vi "MNIST_WB big pattern_LCD_sub.vi"(1 "최소값":dbl=-255.0, 2 "최대값":dbl=255.0, 3 "배열":dbl[][](array[numeric])=[[255.0, 255.0, 255.0, 255.0, 255.0, 255.0, 255.0, 255.0, 255.0, 255.0, 255.0, 255.0, 255.0, 255.0, 255.0, 255.0, 255.0, 255.0, 255.0, 255.0, 255.0, 255.0, 255.0, 255.0, 255.0, 255.0, 255.0, 255.0], [255.0, 255.0, 255.0, 255.0, 255.0, 255.0, 255.0, 255.0, 255.0, 255.0, 255.0, 255.0, 255.0, 255.0, 255.0, 255.0, 255.0, 255.0, 255.0, 255.0, 255.0, 255.0, 255.0, 255.0, 255.0, 255.0, 255.0, 255.0], [255.0, 255.0, 255.0, 255.0, 255.0, 255.0, 255.0, 255.0, 255.0, 255.0, 255.0, 255.0, 255.0, 255.0, 255.0, 255.0, 255.0, 255.0, 255.0, 255.0, 255.0, 255.0, 255.0, 255.0, 255.0, 255.0, 255.0, 255.0], [255.0, 255.0, 255.0, 255.0, 255.0, 255.0, 255.0, 255.0, 255.0, 255.0, 255.0, 255.0, 255.0, 255.0, 255.0, 255.0, 255.0, 255.0, 255.0, 255.0, 255.0, 255.0, 255.0, 255.0, 255.0, 255.0, 255.0, 255.0], [255.0, 255.0, 255.0, 255.0, 255.0, 255.0, 255.0, 255.0, 255.0, 255.0, 255.0, 255.0, 255.0, 255.0, 255.0, 255.0, 255.0, 255.0, 255.0, 255.0, 255.0, 255.0, 255.0, 255.0, 255.0, 255.0, 255.0, 255.0], [255.0, 255.0, 255.0, 255.0, 255.0, 255.0, 255.0, 255.0, 255.0, 255.0, 255.0, 255.0, 255.0, 255.0, 255.0, 255.0, 255.0, 255.0, 255.0, 255.0, 255.0, 255.0, 255.0, 255.0, 255.0, 255.0, 255.0, 255.0], [255.0, 255.0, 255.0, 255.0, 255.0, 255.0, 255.0, 255.0, 255.0, 255.0, 255.0, 255.0, 255.0, 255.0, 255.0, 255.0, 255.0, 255.0, 255.0, 255.0, 255.0, 255.0, 255.0, 255.0, 255.0, 255.0, 255.0, 255.0], [255.0, 255.0, 255.0, 255.0, 255.0, 255.0, 255.0, 255.0, 255.0, 255.0, 255.0, 255.0, 255.0, 255.0, 255.0, 255.0, 255.0, 255.0, 255.0, 255.0, 255.0, 255.0, 255.0, 255.0, 255.0, 255.0, 255.0, 255.0], [255.0, 255.0, 255.0, 255.0, 255.0, 255.0, 255.0, 255.0, 255.0, 255.0, 255.0, 255.0, 255.0, 255.0, 255.0, 255.0, 255.0, 255.0, 255.0, 255.0, 255.0, 255.0, 255.0, 255.0, 255.0, 255.0, 255.0, 255.0], [255.0, 255.0, 255.0, 255.0, 255.0, 255.0, 255.0, 255.0, 255.0, 255.0, 255.0, 255.0, 255.0, 255.0, 255.0, 255.0, 255.0, 255.0, 255.0, 255.0, 255.0, 255.0, 255.0, 255.0, 255.0, 255.0, 255.0, 255.0], [255.0, 255.0, 255.0, 255.0, 255.0, 255.0, 255.0, 255.0, 255.0, 255.0, 255.0, 255.0, 255.0, 255.0, 255.0, 255.0, 255.0, 255.0, 255.0, 255.0, 255.0, 255.0, 255.0, 255.0, 255.0, 255.0, 255.0, 255.0], [255.0, 255.0, 255.0, 255.0, 255.0, 255.0, 255.0, 255.0, 255.0, 255.0, 255.0, 255.0, 255.0, 255.0, 255.0, 255.0, 255.0, 255.0, 255.0, 255.0, 255.0, 255.0, 255.0, 255.0, 255.0, 255.0, 255.0, 255.0], [255.0, 255.0, 255.0, 255.0, 255.0, 255.0, 255.0, 255.0, 255.0, 255.0, 255.0, 255.0, 255.0, 255.0, 255.0, 255.0, 255.0, 255.0, 255.0, 255.0, 255.0, 255.0, 255.0, 255.0, 255.0, 255.0, 255.0, 255.0], [255.0, 255.0, 255.0, 255.0, 255.0, 255.0, 255.0, 255.0, 255.0, 255.0, 255.0, 255.0, 255.0, 255.0, 255.0, 255.0, 255.0, 255.0, 255.0, 255.0, 255.0, 255.0, 255.0, 255.0, 255.0, 255.0, 255.0, 255.0], [255.0, 255.0, 255.0, 255.0, 255.0, 255.0, 255.0, 255.0, 255.0, 255.0, 255.0, 255.0, 255.0, 255.0, 255.0, 255.0, 255.0, 255.0, 255.0, 255.0, 255.0, 255.0, 255.0, 255.0, 255.0, 255.0, 255.0, 255.0], [255.0, 255.0, 255.0, 255.0, 255.0, 255.0, 255.0, 255.0, 255.0, 255.0, 255.0, 255.0, 255.0, 255.0, 255.0, 255.0, 255.0, 255.0, 255.0, 255.0, 255.0, 255.0, 255.0, 255.0, 255.0, 255.0, 255.0, 255.0], [255.0, 255.0, 255.0, 255.0, 255.0, 255.0, 255.0, 255.0, 255.0, 255.0, 255.0, 255.0, 255.0, 255.0, 255.0, 255.0, 255.0, 255.0, 255.0, 255.0, 255.0, 255.0, 255.0, 255.0, 255.0, 255.0, 255.0, 255.0], [255.0, 255.0, 255.0, 255.0, 255.0, 255.0, 255.0, 255.0, 255.0, 255.0, 255.0, 255.0, 255.0, 255.0, 255.0, 255.0, 255.0, 255.0, 255.0, 255.0, 255.0, 255.0, 255.0, 255.0, 255.0, 255.0, 255.0, 255.0], [255.0, 255.0, 255.0, 255.0, 255.0, 255.0, 255.0, 255.0, 255.0, 255.0, 255.0, 255.0, 255.0, 255.0, 255.0, 255.0, 255.0, 255.0, 255.0, 255.0, 255.0, 255.0, 255.0, 255.0, 255.0, 255.0, 255.0, 255.0], [255.0, 255.0, 255.0, 255.0, 255.0, 255.0, 255.0, 255.0, 255.0, 255.0, 255.0, 255.0, 255.0, 255.0, 255.0, 255.0, 255.0, 255.0, 255.0, 255.0, 255.0, 255.0, 255.0, 255.0, 255.0, 255.0, 255.0, 255.0], [255.0, 255.0, 255.0, 255.0, 255.0, 255.0, 255.0, 255.0, 255.0, 255.0, 255.0, 255.0, 255.0, 255.0, 255.0, 255.0, 255.0, 255.0, 255.0, 255.0, 255.0, 255.0, 255.0, 255.0, 255.0, 255.0, 255.0, 255.0], [255.0, 255.0, 255.0, 255.0, 255.0, 255.0, 255.0, 255.0, 255.0, 255.0, 255.0, 255.0, 255.0, 255.0, 255.0, 255.0, 255.0, 255.0, 255.0, 255.0, 255.0, 255.0, 255.0, 255.0, 255.0, 255.0, 255.0, 255.0], [255.0, 255.0, 255.0, 255.0, 255.0, 255.0, 255.0, 255.0, 255.0, 255.0, 255.0, 255.0, 255.0, 255.0, 255.0, 255.0, 255.0, 255.0, 255.0, 255.0, 255.0, 255.0, 255.0, 255.0, 255.0, 255.0, 255.0, 255.0], [255.0, 255.0, 255.0, 255.0, 255.0, 255.0, 255.0, 255.0, 255.0, 255.0, 255.0, 255.0, 255.0, 255.0, 255.0, 255.0, 255.0, 255.0, 255.0, 255.0, 255.0, 255.0, 255.0, 255.0, 255.0, 255.0, 255.0, 255.0], [255.0, 255.0, 255.0, 255.0, 255.0, 255.0, 255.0, 255.0, 255.0, 255.0, 255.0, 255.0, 255.0, 255.0, 255.0, 255.0, 255.0, 255.0, 255.0, 255.0, 255.0, 255.0, 255.0, 255.0, 255.0, 255.0, 255.0, 255.0], [255.0, 255.0, 255.0, 255.0, 255.0, 255.0, 255.0, 255.0, 255.0, 255.0, 255.0, 255.0, 255.0, 255.0, 255.0, 255.0, 255.0, 255.0, 255.0, 255.0, 255.0, 255.0, 255.0, 255.0, 255.0, 255.0, 255.0, 255.0], [255.0, 255.0, 255.0, 255.0, 255.0, 255.0, 255.0, 255.0, 255.0, 255.0, 255.0, 255.0, 255.0, 255.0, 255.0, 255.0, 255.0, 255.0, 255.0, 255.0, 255.0, 255.0, 255.0, 255.0, 255.0, 255.0, 255.0, 255.0], [255.0, 255.0, 255.0, 255.0, 255.0, 255.0, 255.0, 255.0, 255.0, 255.0, 255.0, 255.0, 255.0, 255.0, 255.0, 255.0, 255.0, 255.0, 255.0, 255.0, 255.0, 255.0, 255.0, 255.0, 255.0, 255.0, 255.0, 255.0], [0.0, 0.0, 0.0, 0.0, 0.0, 0.0, 0.0, 0.0, 0.0, 0.0, 0.0, 0.0, 0.0, 0.0, 0.0, 0.0, 0.0, 0.0, 0.0, 0.0, 0.0, 0.0, 0.0, 0.0, 0.0, 0.0, 0.0, 0.0]]) -> (0 "MNIST_Input":dbl[][](graph)=[[255.0, 255.0, 255.0, 255.0, 255.0, 255.0, 255.0, 255.0, 255.0, 255.0, 255.0, 255.0, 255.0, 255.0, 255.0, 255.0, 255.0, 255.0, 255.0, 255.0, 255.0, 255.0, 255.0, 255.0, 255.0, 255.0, 255.0, 255.0], [255.0, 255.0, 255.0, 255.0, 255.0, 255.0, 255.0, 255.0, 255.0, 255.0, 255.0, 255.0, 255.0, 255.0, 255.0, 255.0, 255.0, 255.0, 255.0, 255.0, 255.0, 255.0, 255.0, 255.0, 255.0, 255.0, 255.0, 255.0], [255.0, 255.0, 255.0, 255.0, 255.0, 255.0, 255.0, 255.0, 255.0, 255.0, 255.0, 255.0, 255.0, 255.0, 255.0, 255.0, 255.0, 255.0, 255.0, 255.0, 255.0, 255.0, 255.0, 255.0, 255.0, 255.0, 255.0, 255.0], [255.0, 255.0, 255.0, 255.0, 255.0, 255.0, 255.0, 255.0, 255.0, 255.0, 255.0, 255.0, 255.0, 255.0, 255.0, 255.0, 255.0, 255.0, 255.0, 255.0, 255.0, 255.0, 255.0, 255.0, 255.0, 255.0, 255.0, 255.0], [255.0, 255.0, 255.0, 255.0, 255.0, 255.0, 255.0, 255.0, 255.0, 255.0, 255.0, 255.0, 255.0, 255.0, 255.0, 255.0, 255.0, 255.0, 255.0, 255.0, 255.0, 255.0, 255.0, 255.0, 255.0, 255.0, 255.0, 255.0], [255.0, 255.0, 255.0, 255.0, 255.0, 255.0, 255.0, 255.0, 255.0, 255.0, 255.0, 255.0, 255.0, 255.0, 255.0, 255.0, 255.0, 255.0, 255.0, 255.0, 255.0, 255.0, 255.0, 255.0, 255.0, 255.0, 255.0, 255.0], [255.0, 255.0, 255.0, 255.0, 255.0, 255.0, 255.0, 255.0, 255.0, 255.0, 255.0, 255.0, 255.0, 255.0, 255.0, 255.0, 255.0, 255.0, 255.0, 255.0, 255.0, 255.0, 255.0, 255.0, 255.0, 255.0, 255.0, 255.0], [255.0, 255.0, 255.0, 255.0, 255.0, 255.0, 255.0, 255.0, 255.0, 255.0, 255.0, 255.0, 255.0, 255.0, 255.0, 255.0, 255.0, 255.0, 255.0, 255.0, 255.0, 255.0, 255.0, 255.0, 255.0, 255.0, 255.0, 255.0], [255.0, 255.0, 255.0, 255.0, 255.0, 255.0, 255.0, 255.0, 255.0, 255.0, 255.0, 255.0, 255.0, 255.0, 255.0, 255.0, 255.0, 255.0, 255.0, 255.0, 255.0, 255.0, 255.0, 255.0, 255.0, 255.0, 255.0, 255.0], [255.0, 255.0, 255.0, 255.0, 255.0, 255.0, 255.0, 255.0, 255.0, 255.0, 255.0, 255.0, 255.0, 255.0, 255.0, 255.0, 255.0, 255.0, 255.0, 255.0, 255.0, 255.0, 255.0, 255.0, 255.0, 255.0, 255.0, 255.0], [255.0, 255.0, 255.0, 255.0, 255.0, 255.0, 255.0, 255.0, 255.0, 255.0, 255.0, 255.0, 255.0, 255.0, 255.0, 255.0, 255.0, 255.0, 255.0, 255.0, 255.0, 255.0, 255.0, 255.0, 255.0, 255.0, 255.0, 255.0], [255.0, 255.0, 255.0, 255.0, 255.0, 255.0, 255.0, 255.0, 255.0, 255.0, 255.0, 255.0, 255.0, 255.0, 255.0, 255.0, 255.0, 255.0, 255.0, 255.0, 255.0, 255.0, 255.0, 255.0, 255.0, 255.0, 255.0, 255.0], [255.0, 255.0, 255.0, 255.0, 255.0, 255.0, 255.0, 255.0, 255.0, 255.0, 255.0, 255.0, 255.0, 255.0, 255.0, 255.0, 255.0, 255.0, 255.0, 255.0, 255.0, 255.0, 255.0, 255.0, 255.0, 255.0, 255.0, 255.0], [255.0, 255.0, 255.0, 255.0, 255.0, 255.0, 255.0, 255.0, 255.0, 255.0, 255.0, 255.0, 255.0, 255.0, 255.0, 255.0, 255.0, 255.0, 255.0, 255.0, 255.0, 255.0, 255.0, 255.0, 255.0, 255.0, 255.0, 255.0], [255.0, 255.0, 255.0, 255.0, 255.0, 255.0, 255.0, 255.0, 255.0, 255.0, 255.0, 255.0, 255.0, 255.0, 255.0, 255.0, 255.0, 255.0, 255.0, 255.0, 255.0, 255.0, 255.0, 255.0, 255.0, 255.0, 255.0, 255.0], [255.0, 255.0, 255.0, 255.0, 255.0, 255.0, 255.0, 255.0, 255.0, 255.0, 255.0, 255.0, 255.0, 255.0, 255.0, 255.0, 255.0, 255.0, 255.0, 255.0, 255.0, 255.0, 255.0, 255.0, 255.0, 255.0, 255.0, 255.0], [255.0, 255.0, 255.0, 255.0, 255.0, 255.0, 255.0, 255.0, 255.0, 255.0, 255.0, 255.0, 255.0, 255.0, 255.0, 255.0, 255.0, 255.0, 255.0, 255.0, 255.0, 255.0, 255.0, 255.0, 255.0, 255.0, 255.0, 255.0], [255.0, 255.0, 255.0, 255.0, 255.0, 255.0, 255.0, 255.0, 255.0, 255.0, 255.0, 255.0, 255.0, 255.0, 255.0, 255.0, 255.0, 255.0, 255.0, 255.0, 255.0, 255.0, 255.0, 255.0, 255.0, 255.0, 255.0, 255.0], [255.0, 255.0, 255.0, 255.0, 255.0, 255.0, 255.0, 255.0, 255.0, 255.0, 255.0, 255.0, 255.0, 255.0, 255.0, 255.0, 255.0, 255.0, 255.0, 255.0, 255.0, 255.0, 255.0, 255.0, 255.0, 255.0, 255.0, 255.0], [255.0, 255.0, 255.0, 255.0, 255.0, 255.0, 255.0, 255.0, 255.0, 255.0, 255.0, 255.0, 255.0, 255.0, 255.0, 255.0, 255.0, 255.0, 255.0, 255.0, 255.0, 255.0, 255.0, 255.0, 255.0, 255.0, 255.0, 255.0], [255.0, 255.0, 255.0, 255.0, 255.0, 255.0, 255.0, 255.0, 255.0, 255.0, 255.0, 255.0, 255.0, 255.0, 255.0, 255.0, 255.0, 255.0, 255.0, 255.0, 255.0, 255.0, 255.0, 255.0, 255.0, 255.0, 255.0, 255.0], [255.0, 255.0, 255.0, 255.0, 255.0, 255.0, 255.0, 255.0, 255.0, 255.0, 255.0, 255.0, 255.0, 255.0, 255.0, 255.0, 255.0, 255.0, 255.0, 255.0, 255.0, 255.0, 255.0, 255.0, 255.0, 255.0, 255.0, 255.0], [255.0, 255.0, 255.0, 255.0, 255.0, 255.0, 255.0, 255.0, 255.0, 255.0, 255.0, 255.0, 255.0, 255.0, 255.0, 255.0, 255.0, 255.0, 255.0, 255.0, 255.0, 255.0, 255.0, 255.0, 255.0, 255.0, 255.0, 255.0], [255.0, 255.0, 255.0, 255.0, 255.0, 255.0, 255.0, 255.0, 255.0, 255.0, 255.0, 255.0, 255.0, 255.0, 255.0, 255.0, 255.0, 255.0, 255.0, 255.0, 255.0, 255.0, 255.0, 255.0, 255.0, 255.0, 255.0, 255.0], [255.0, 255.0, 255.0, 255.0, 255.0, 255.0, 255.0, 255.0, 255.0, 255.0, 255.0, 255.0, 255.0, 255.0, 255.0, 255.0, 255.0, 255.0, 255.0, 255.0, 255.0, 255.0, 255.0, 255.0, 255.0, 255.0, 255.0, 255.0], [255.0, 255.0, 255.0, 255.0, 255.0, 255.0, 255.0, 255.0, 255.0, 255.0, 255.0, 255.0, 255.0, 255.0, 255.0, 255.0, 255.0, 255.0, 255.0, 255.0, 255.0, 255.0, 255.0, 255.0, 255.0, 255.0, 255.0, 255.0], [255.0, 255.0, 255.0, 255.0, 255.0, 255.0, 255.0, 255.0, 255.0, 255.0, 255.0, 255.0, 255.0, 255.0, 255.0, 255.0, 255.0, 255.0, 255.0, 255.0, 255.0, 255.0, 255.0, 255.0, 255.0, 255.0, 255.0, 255.0], [255.0, 255.0, 255.0, 255.0, 255.0, 255.0, 255.0, 255.0, 255.0, 255.0, 255.0, 255.0, 255.0, 255.0, 255.0, 255.0, 255.0, 255.0, 255.0, 255.0, 255.0, 255.0, 255.0, 255.0, 255.0, 255.0, 255.0, 255.0], [0.0, 0.0, 0.0, 0.0, 0.0, 0.0, 0.0, 0.0, 0.0, 0.0, 0.0, 0.0, 0.0, 0.0, 0.0, 0.0, 0.0, 0.0, 0.0, 0.0, 0.0, 0.0, 0.0, 0.0, 0.0, 0.0, 0.0, 0.0]])   [LabVIEW 2021]
panel:
  in  "색선택 3":u32[](array[colorbox])=[255, 0, 255]
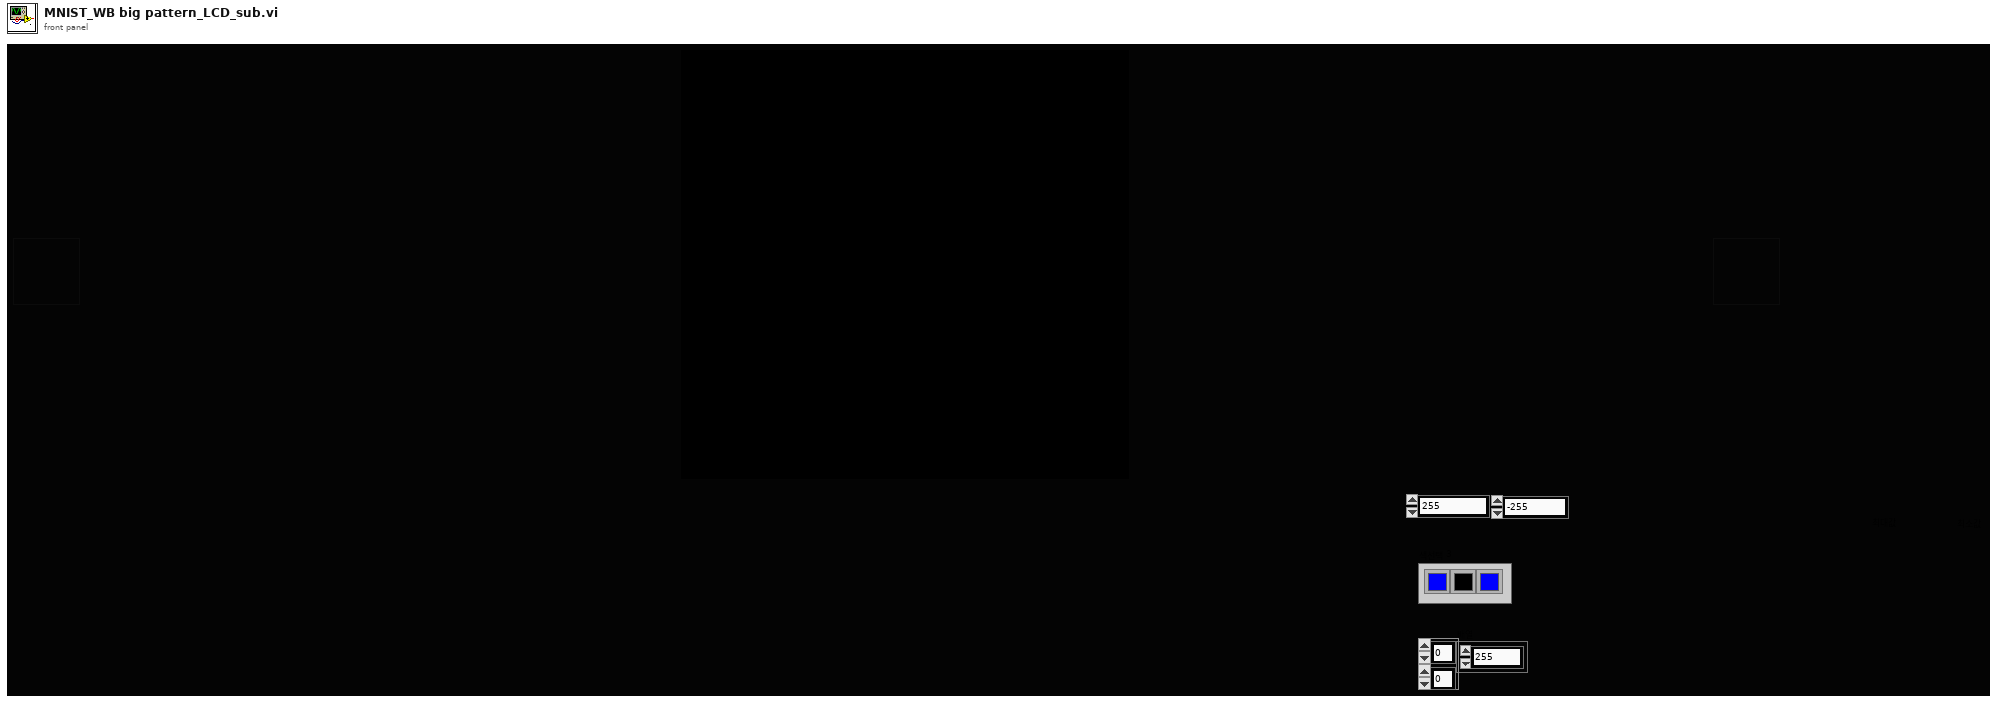
[diagram p1: front panel]
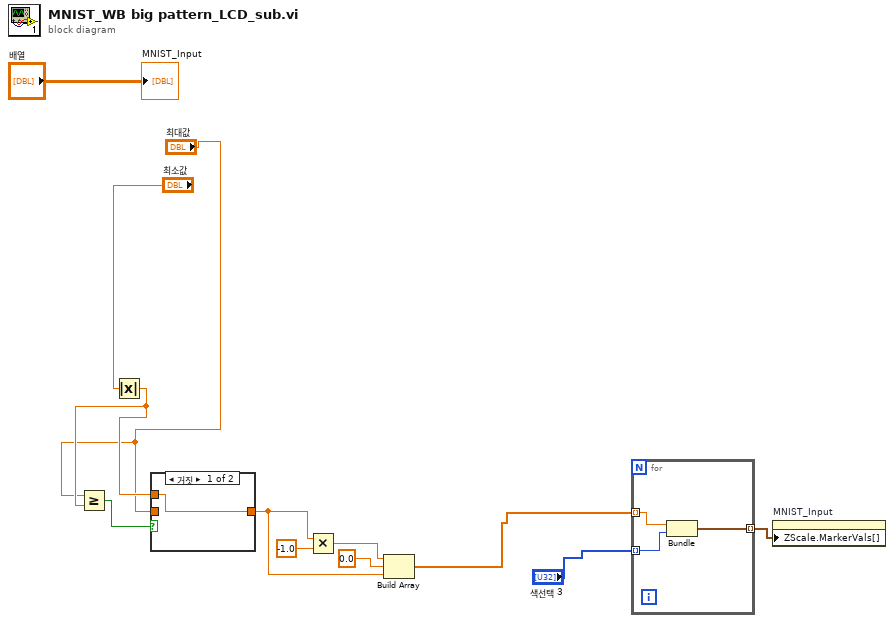
[diagram p0: block diagram]
diagram:
  n1 = Absolute Value(x="최소값") -> (abs(x)=w5:dbl)
  n2 = Greater Or Equal?(x="최대값", y=w5) -> (x >= y?=w11:bool)
  n3 = case shown="거짓" w11 {
    tunnel: "최대값" -> [_ w14]
    tunnel: [w13 w14] -> w7
    tunnel: w5 -> [w13 _]
    frame False {
    }
    frame True {
    }
  }
  n4 = Multiply(x=w7, y=-1.0) -> (x*y=w8:dbl)
  n5 = Build Array(w8, 0.0 ("원소"), w7) -> (w6:dbl[])
  n6 = for {
    tunnel: w6 -> [w17] mode=indexing
    tunnel: "색선택 3" -> [w16] mode=indexing
    tunnel: [w15] -> w3 mode=indexing
    n7 = Bundle("최대값"=w17, "색 상자"=w16) -> (w15:cluster{"최대값":dbl, "색 상자":u32})  [unwired: 1 in]
  }
  n8 = property on="MNIST_Input" class="IntGraph (엄격한)"("ZScale.MarkerVals[]"=w3) -> ()  [unwired: 2 in, 2 out]
  "MNIST_Input" <- "배열"
